vi "Flywheel_Logic_Unit_Test.vi"() -> ()   [LabVIEW 2019]
panel:
  out "RPM output":dbl
  in  "array":dbl[][](array[numeric])
  in  "search_value":ext
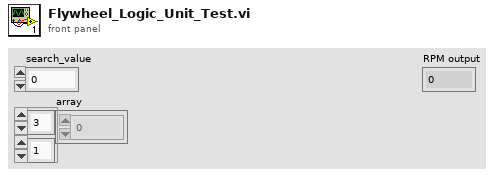
[diagram p1: front panel]
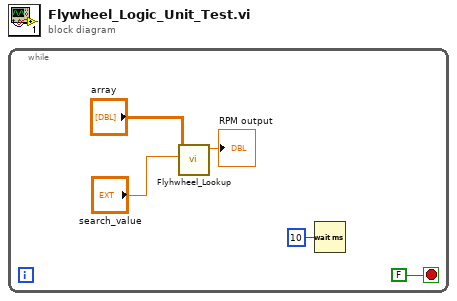
[diagram p0: block diagram]
diagram:
  n1 = while {
    stop <- FALSE stop-if-true
    n2 = call "Flyhwheel_Lookup.vi"("search_value"="search_value", "array"="array") -> ("RPM output"=→"RPM output":dbl)  [unwired: 9 in]
    n3 = Wait (ms)(milliseconds to wait=u32 10) -> ()  [unwired: 1 out]
  }
